vi "Measurement Logic.vi"() -> ()   [LabVIEW 2021, in "Short-Circuit.lvlib"]
uses:
  Short-Circuit.lvlib
  <instrlib>/niDCPower/nidcpower.llb/niDCPower Source Mode.ctl
  <instrlib>/niDCPower/nidcpower.llb/niDCPower Wait For Event - Event.ctl
  <instrlib>/niDCPower/nidcpower.llb/niDCPower Get Channel Name From String.vi
  Controls/LED_SCT_Data.ctl
  <instrlib>/niSwitch/niSwitch.llb/niSwitch Relay Action.ctl
  <instrlib>/niDMM/nidmm.llb/niDMM Function.ctl
  <instrlib>/niDMM/nidmm.llb/niDMM Configure Measurement Digits.vi
  <instrlib>/niDCPower/nidcpower.llb/niDCPower Output Function.ctl
  Measurement Results.ctl
  <instrlib>/niDCPower/nidcpower.llb/niDCPower Configure Digital Edge Source Trigger With Channels.vi
  <instrlib>/niDCPower/nidcpower.llb/niDCPower Configure Digital Edge Measure Trigger With Channels.vi
  <vilib>/Plug-In SDKs/Measurements/Measure Call Context/Measure Call Context.lvclass
  Measurement Configuration.ctl
panel:
  out "measurement results":T1={"Status"="Empty", "Source voltages"=[0.0], "Load voltages"=[0.0], "Source Current"=[0.0], "Load Current"=[0.0]}
  in  "measurement configuration":T2={"DUT setup time"=0.5, "Source delay"=0.5, "Aperture time"=0.5, "Source resource name"="Lorem ipsum dolor sit", "Source sense"=64, "Source current limit"=2.0, "Source maximum power"=20.0, "Source Voltage (Vo)"=3.5, "Load resource name"="", "Load sense"=-64, "Load voltage limit range"=60.0, "Load Voltage Limit"=6.0, "Load Current Level (Io)"=0.1, "Switch resource name"="", "Switch - Load Relay Name"="", "Switch - DMM Relay Name"="", "Relay Topology"="Configured Topology", "DMM resource name"="", "DMM Current Range(A)"=3.0, "SC - Trigger Delay (sec)"=5.0, "SC - Hold Delay (sec)"=5.0, "Resolution in Digits"=6.5} {"Resolution in Digits" items=["3 1/2"=3.5, "4 1/2"=4.5, "5 1/2"=5.5, "6 1/2"=6.5, "7 1/2"=7.5]; "Load Current Level (Io)" format="%.3f"; "Source Voltage (Vo)" format="%.2f"; "Load sense" items=["Local"=1008, "Remote"=1009]; "Source sense" items=["Local"=1008, "Remote"=1009]; "Aperture time" format="%#_6p"; "Source delay" format="%#_6p"; "DUT setup time" format="%#_6p"}
  out "measure call context out":refnum<class "Measure Call Context.lvclass">
  in  "measure call context in":refnum<class "Measure Call Context.lvclass">
  out "error out":errorcluster
  in  "error in":errorcluster
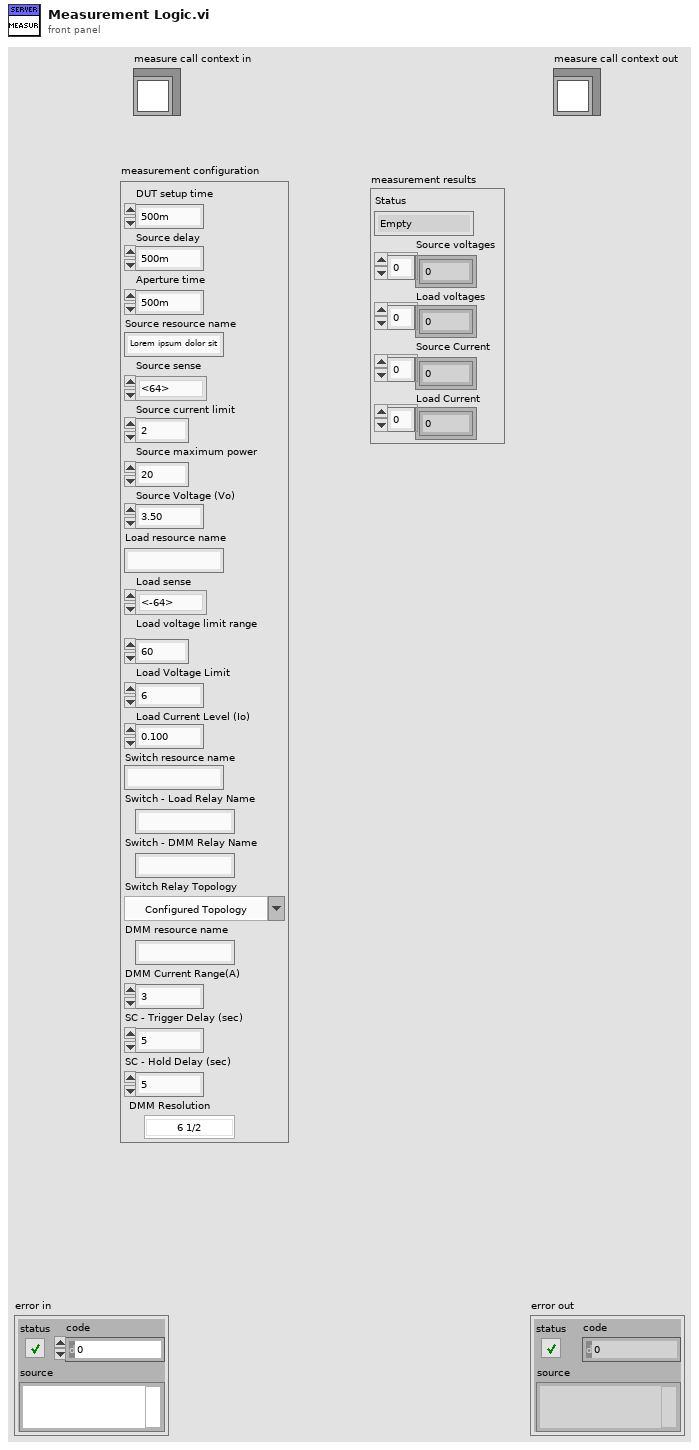
[diagram p1: front panel]
types:
  T1 = typedef "Short-Circuit.lvlib/Measurement Results.ctl" = cluster{"Status":string, "Source voltages":dbl[], "Load voltages":dbl[], "Source Current":dbl[], "Load Current":dbl[]}
  T2 = typedef "Short-Circuit.lvlib/Measurement Configuration.ctl" = cluster{"DUT setup time":dbl, "Source delay":dbl, "Aperture time":dbl, "Source resource name":string, "Source sense":i32, "Source current limit":dbl, "Source maximum power":dbl, "Source Voltage (Vo)":dbl, "Load resource name":string, "Load sense":i32, "Load voltage limit range":dbl, "Load Voltage Limit":dbl, "Load Current Level (Io)":dbl, "Switch resource name":string, "Switch - Load Relay Name":string, "Switch - DMM Relay Name":string, "Relay Topology":string, "DMM resource name":string, "DMM Current Range(A)":dbl, "SC - Trigger Delay (sec)":dbl, "SC - Hold Delay (sec)":dbl, "Resolution in Digits":dbl}
  T3 = typedef "Short-Circuit.lvlib/LED_SCT_Data.ctl" = cluster{"Load channel name":string, "Load out":refnum<k15>, "Source out":refnum<k15>, "Source channel name":string, "Source sequence name":string, "Source terminal name":string, "Measure terminal name":string, "Load Voltage-out":dbl[], "Load Current - out":dbl[], "Source Voltage-out":dbl[], "Source Current - out":dbl[], "Load Relay name":string, "DMM Relay name":string, "Switch out":refnum<k15>, "DMM out":refnum<k15>, "measurement results":T1, "SCT Completed?":bool, "DMM Current Reading":dbl}
  T4 = typedef "niDMM Function.ctl" = enum16{"DC Volts", "AC Volts", "DC Current", "AC Current", "2-wire Resistance", "4-wire Resistance", "Diode", "Frequency", "Period", "AC Volts DC Coupled", "Capacitance", "Inductance", "Temperature"}
  T5 = typedef "niDCPower Wait For Event - Event.ctl" = i32
  T6 = typedef "niDCPower Source Mode.ctl" = i32
  T7 = typedef "niSwitch Relay Action.ctl" = i32
  T8 = typedef "niDCPower Output Function.ctl" = i32
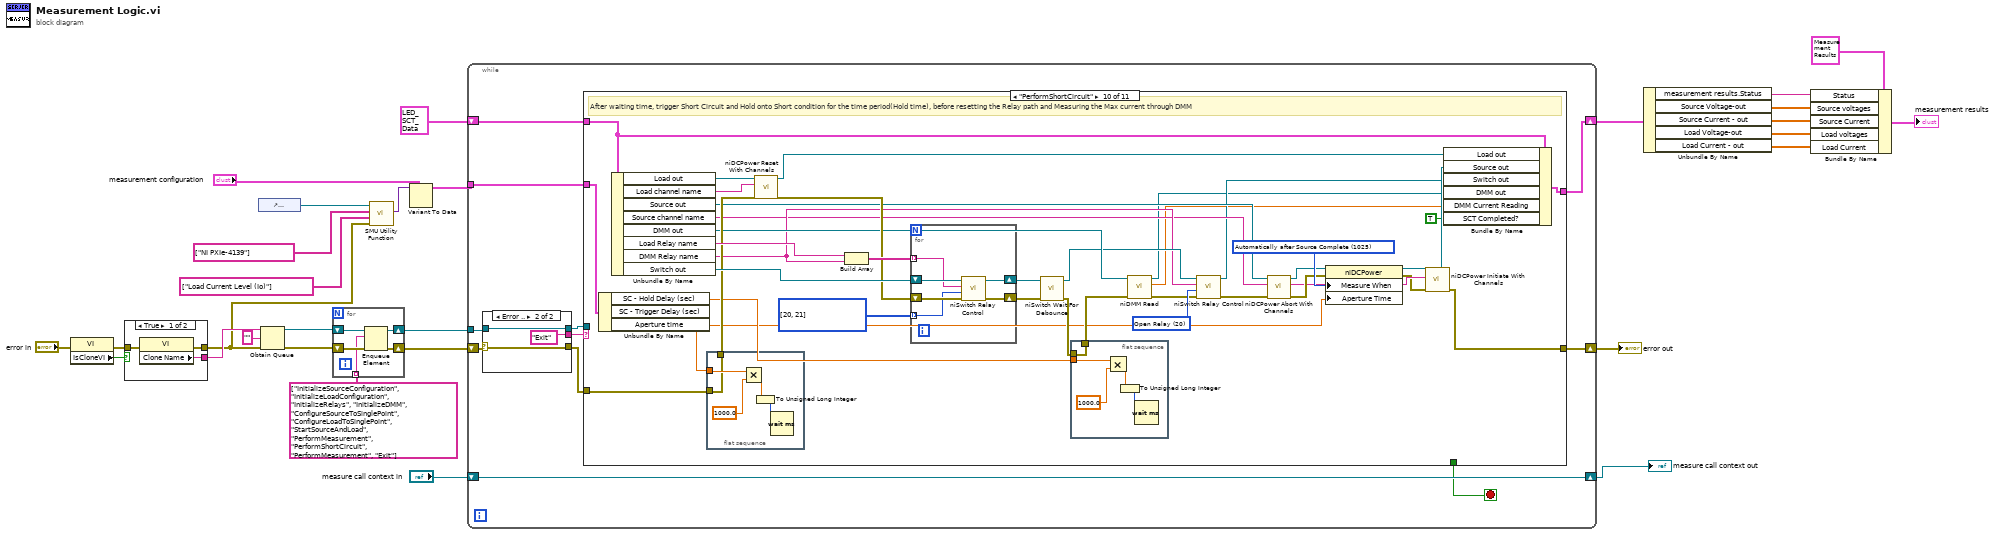
[diagram p0: block diagram]
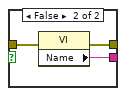
[diagram p2: hidden frame]
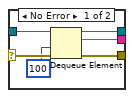
[diagram p3: hidden frame]
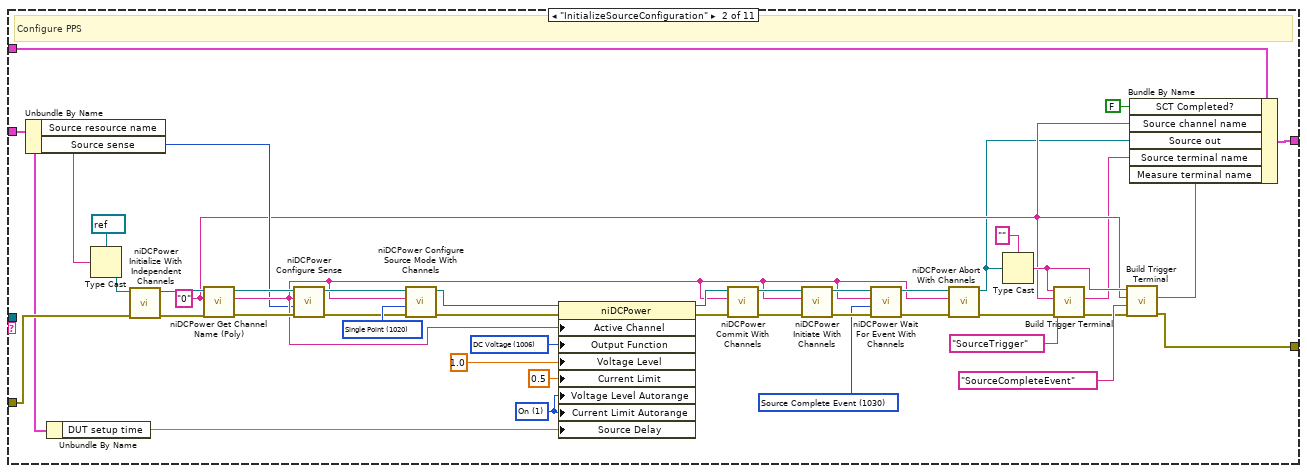
[diagram p5: hidden frame]
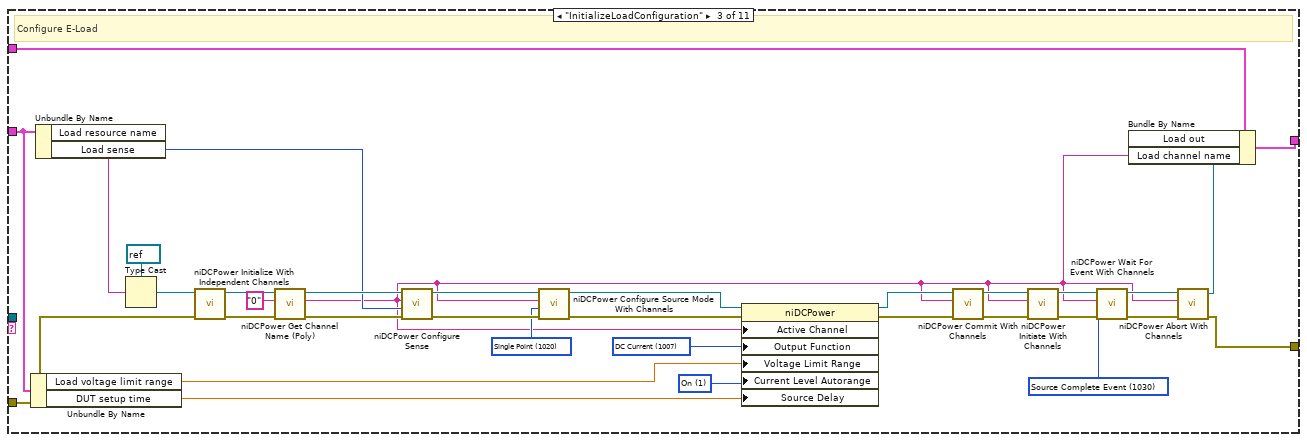
[diagram p6: hidden frame]
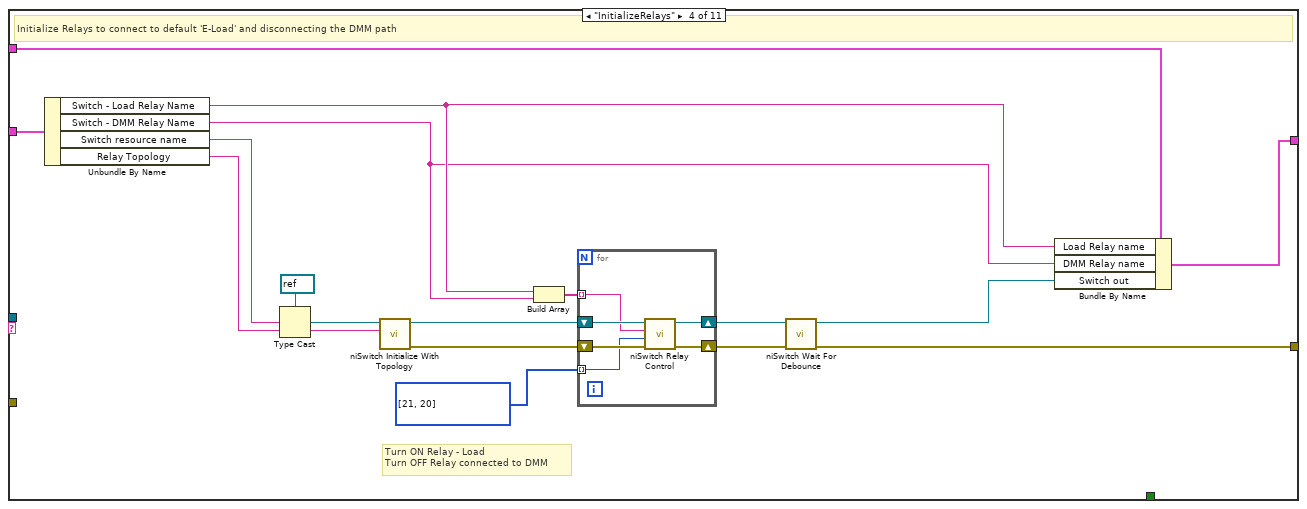
[diagram p7: hidden frame]
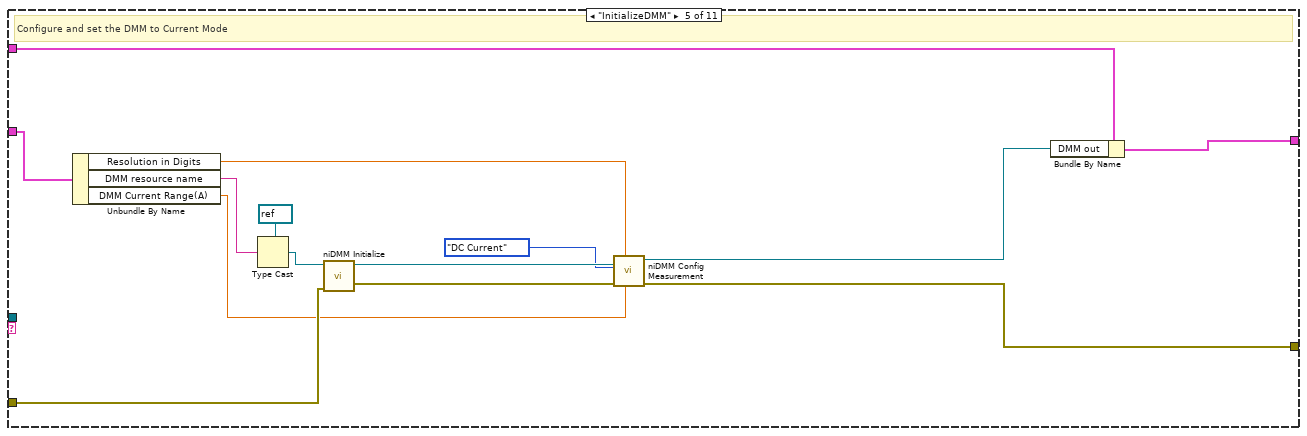
[diagram p8: hidden frame]
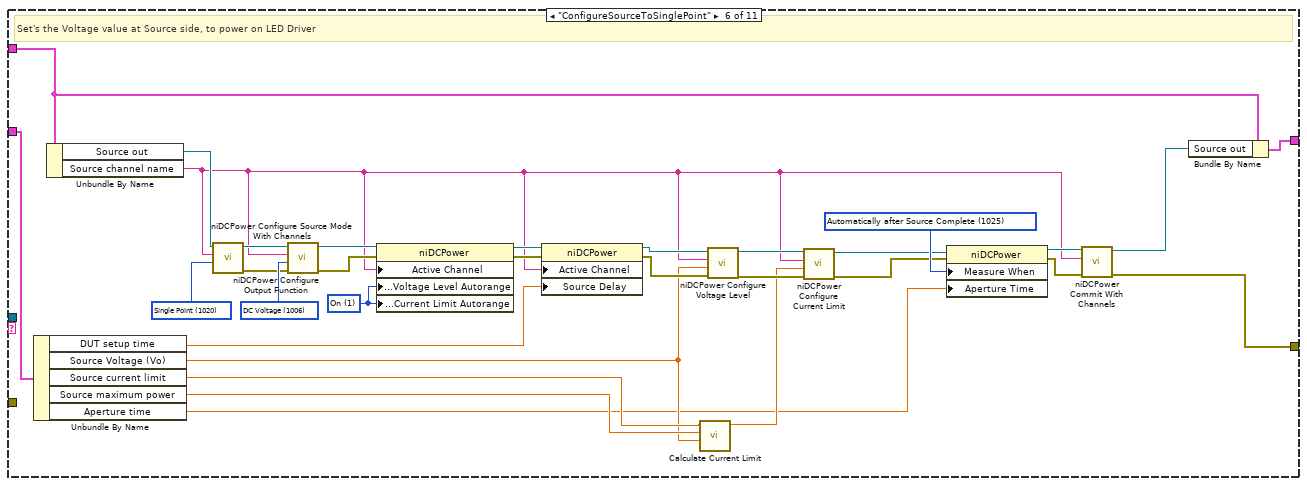
[diagram p9: hidden frame]
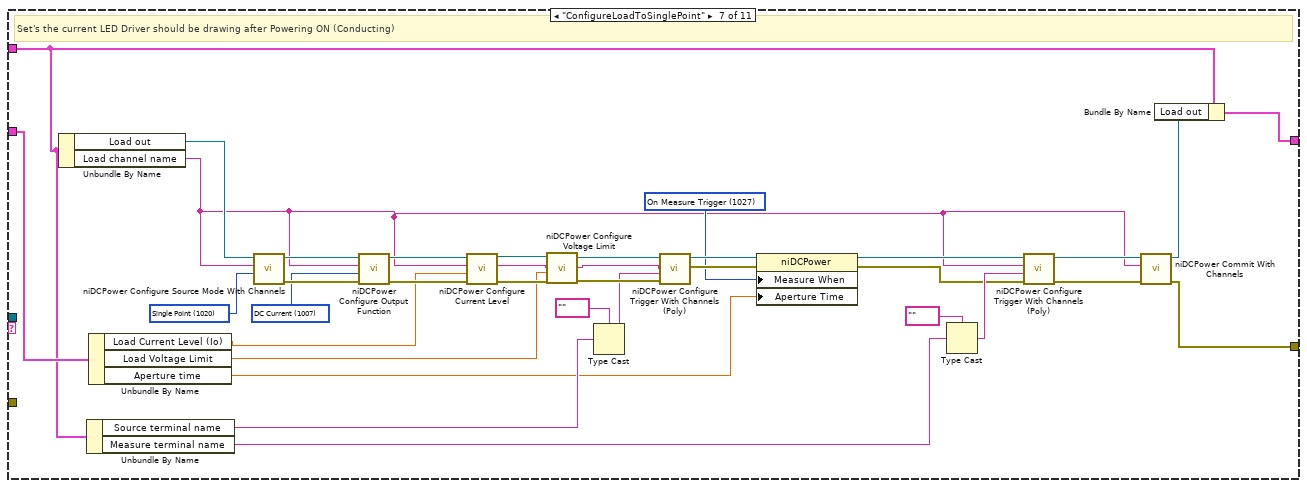
[diagram p10: hidden frame]
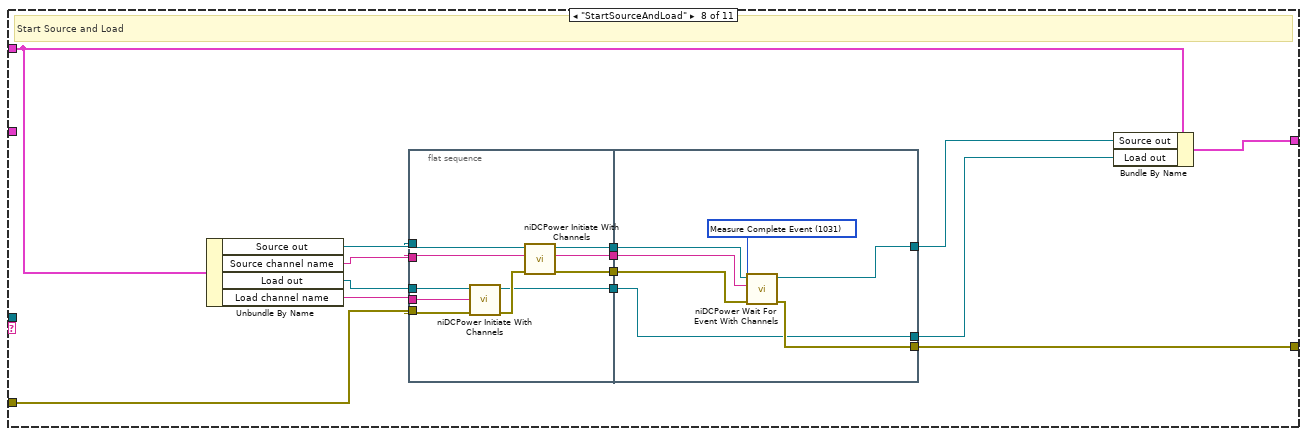
[diagram p11: hidden frame]
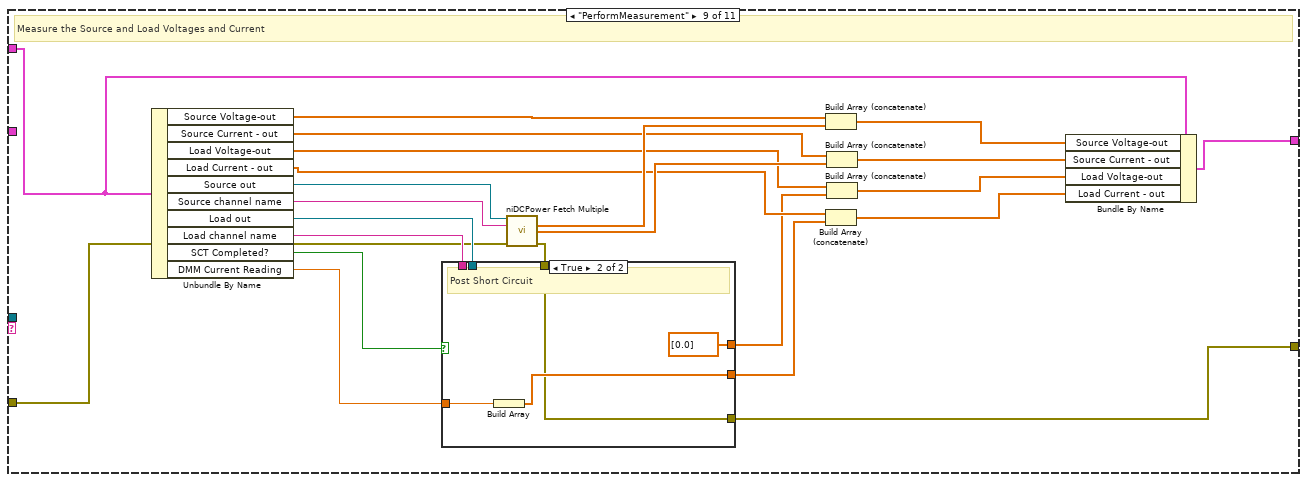
[diagram p12: hidden frame]
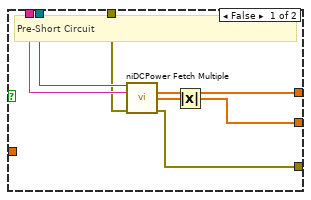
[diagram p13: hidden frame]
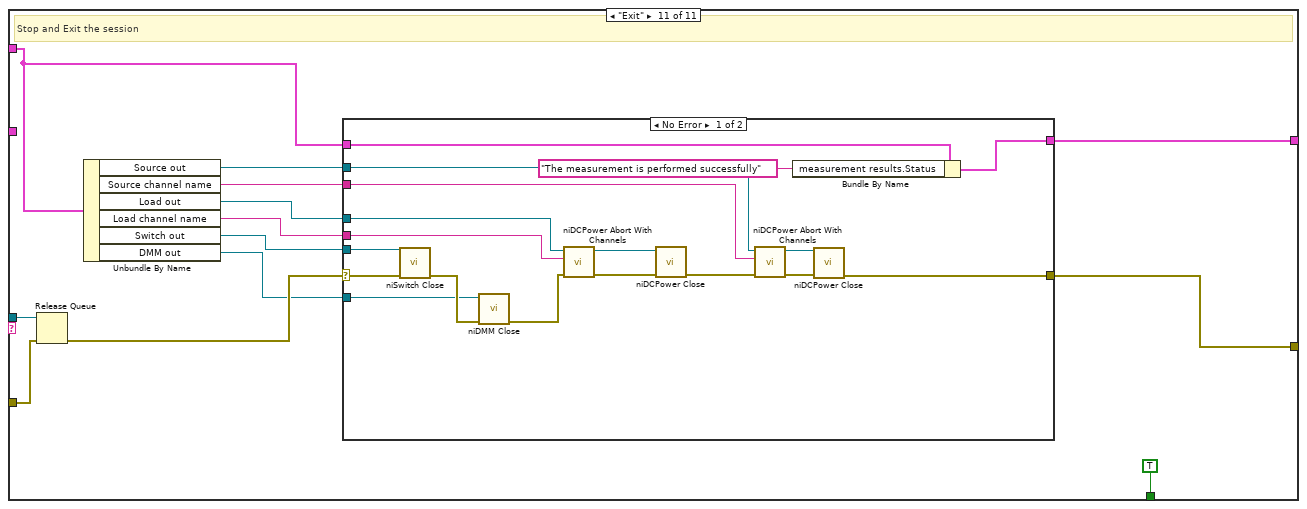
[diagram p14: hidden frame]
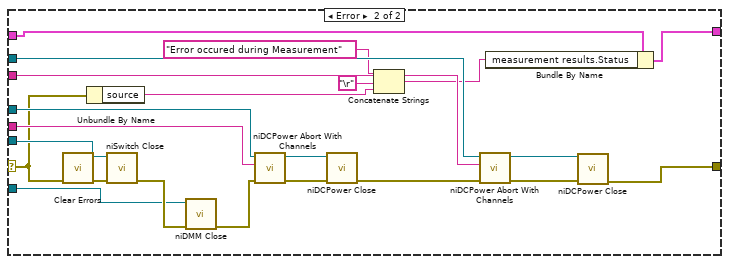
[diagram p15: hidden frame]
diagram:
  n1 = property class="VI"(error in="error in") -> (error out=w28:errorcluster, "IsCloneVI"=w29:bool)  [unwired: 1 in, 1 out]
  n2 = case shown="True" w29 {
    tunnel: [w32 w35] -> w4
    tunnel: [w31 w34] -> w23
    tunnel: w28 -> [w30 w33]
    frame True {
      n3 = property class="VI"(error in=w30) -> (error out=w32:errorcluster, "Clone Name"=w31:string)  [unwired: 1 in, 1 out]
    }
    frame False {
      n4 = property class="VI"(error in=w33) -> (error out=w35:errorcluster, "Name"=w34:string)  [unwired: 1 in, 1 out]
    }
  }
  n5 = control-ref of="measurement configuration"() -> (w7:refnum<vi>)
  n6 = Obtain Queue(name (unnamed)=w23, element data type="", error in (no error)=w4) -> (queue out=w26:refnum<queue>, error out=w27:errorcluster)  [unwired: 2 in, 1 out]
  n7 = for {
    shift-right: [w38] -> w21
    shift-left: w26 -> [w40]
    shift-right: [w37] -> w22
    shift-left: w27 -> [w39]
    tunnel: string[] ["InitializeSourceConfiguration", "InitializeLoadConfiguration", "InitializeRelays", "InitializeDMM", "ConfigureSourceToSinglePoint", "ConfigureLoadToSinglePoint", "StartSourceAndLoad", "PerformMeasurement", "PerformShortCircuit", "PerformMeasurement", "Exit"] ("Step sequence") -> [w36] mode=indexing
    n8 = Enqueue Element(queue=w40, element=w36, error in (no error)=w39) -> (queue out=w38:refnum<queue>, error out=w37:errorcluster)  [unwired: 1 in, 1 out]
  }
  n9 = call "SMU Utility Function.vi"("error in"=w4, "Load Current Parameters"=string[] ["Load Current Level (Io)"], "SMU Model"=string[] ["NI PXIe-4139"], "Measurement Configuration Ref"=w7) -> ("Measurement Configuration Out"=w3:variant)  [unwired: 6 in, 1 out]
  n10 = Variant To Data(type="measurement configuration", Variant=w3) -> (data=w1:T2)  [unwired: 1 in, 1 out]
  n11 = while {
    tunnel: w21 -> [w51]
    shift-right: [w44] -> w16
    shift-left: w22 -> [w50]
    tunnel: w1 -> [w47]
    shift-right: [w45] -> w15
    shift-left: T3 {"Load channel name"="", "Load out"="", "Source out"="", "Source channel name"="", "Source sequence name"="", "Source terminal name"="", "Measure terminal name"="", "Load Voltage-out"=[], "Load Current - out"=[], "Source Voltage-out"=[], "Source Current - out"=[], "Load Relay name"="", "DMM Relay name"="", "Switch out"="", "DMM out"="", "measurement results"={"Status"="Empty", "Source voltages"=[0.0], "Load voltages"=[0.0], "Source Current"=[0.0], "Load Current"=[0.0]}, "SCT Completed?"=FALSE, "DMM Current Reading"=0.0} ("Cluster") -> [w46]
    shift-right: [w43] -> w17
    shift-left: "measure call context in" -> [w43]
    stop <- w41 stop-if-true
    n12 = case shown="Error .." w50 {
      selector: w50 -> [w55 w59]
      tunnel: w51 -> [w57 w58]
      tunnel: [w56 "Exit" ("t")] -> w48
      tunnel: [w54 w59] -> w49
      tunnel: [w52 w58] -> w42
      frame No Error {
        n13 = Dequeue Element(queue=w57, timeout in ms (-1)=100, error in (no error)=w55) -> (queue out=w52:refnum<queue>, element=w56:string, error out=w54:errorcluster)  [unwired: 1 out]
      }
      frame Error {
      }
    }
    n14 = case shown="\"PerformShortCircuit\"" w48 {
      tunnel: w49 -> [w62 w83 w116 _ w170 _ _ w247 w275 w333 w372]
      tunnel: w47 -> [_ w78 w114 w151 w174 w184 w218 _ _ w334 _]
      tunnel: w46 -> [w61 w72 w112 w146 w167 w189 w212 w246 w281 w342 w370]
      tunnel: [w61 w67 w108 w142 w165 w187 w209 w243 w276 w306 w365] -> w45
      tunnel: [w62 w64 w109 w141 w164 w186 w210 w242 w273 w312 w364] -> w44
      tunnel: w42 -> [_ _ _ _ _ _ _ _ _ _ w373]
      tunnel: [_ _ _ _ _ _ _ _ _ _ TRUE] -> w41
      frame "", Default {
      }
      frame "InitializeSourceConfiguration" {
        w71 = "0" ("index")
        w90 = 1 items=["Off", "On"] ("Source:DC Voltage:Voltage Level Autorange")
        w91 = T5 1030 items=["Source Complete Event"=1030, "Measure Complete Event"=1031, "Sequence Iteration Complete Event"=1032, "Sequence Engine Done Event"=1033, "Pulse Complete Event"=1051, "Ready For Pulse Trigger Event"=1052] ("event")
        w102 = T6 1020 items=["Single Point"=1020, "Sequence"=1021] ("source mode")
        w97 = 1006 items=["DC Voltage"=1006, "DC Current"=1007, "Pulse Voltage"=1049, "Pulse Current"=1050] ("Source:Output Function")
        # "Configure PPS"
        n15 = Unbundle By Name(w78) -> ("Source resource name"=w81:string, "Source sense"=w79:i32)
        n16 = Unbundle By Name(w78) -> ("DUT setup time"=w77:dbl)
        n17 = Type Cast(type=refnum<k15> refnum ("resource name"), x=w81) -> (*(type *) &x=w80:refnum<k15>)
        n18 = call <instrlib>:"niDCPower Initialize With Independent Channels.vi"("error in (no error)"=w83, "resource name"=w80) -> ("error out"=w88:errorcluster, "instrument handle out"=w92:refnum<k15>)  [unwired: 8 in]
        n19 = call-poly <instrlib>:"niDCPower Get Channel Name (Poly).vi"("error in (no error)"=w88, "index"=w71, "instrument handle"=w92) -> ("error out"=w87:errorcluster, "name"=w84:string, "instrument handle out"=w89:refnum<k15>)  [unwired: 6 in]
        n20 = call <instrlib>:"niDCPower Configure Sense.vi"("error in (no error)"=w87, "sense"=w79, "channel name"=w84, "instrument handle"=w89) -> ("error out"=w100:errorcluster, "instrument handle out"=w98:refnum<k15>)  [unwired: 6 in]
        n21 = call <instrlib>:"niDCPower Configure Source Mode With Channels.vi"("error in (no error)"=w100, "source mode"=w102, "channel name"=w84, "instrument handle"=w98) -> ("error out"=w101:errorcluster, "instrument handle out"=w99:refnum<k15>)  [unwired: 6 in]
        n22 = property class="niDCPower"(reference=w99, error in=w101, "Active Channel"=w84, "Output Function"=w97, "Voltage Level"=1.0 ("Source:DC Voltage:Voltage Level"), "Current Limit"=0.5 ("Source:DC Voltage:Current Limit"), "Voltage Level Autorange"=w90, "Current Limit Autorange"=w90, "Source Delay"=w77) -> (reference out=w103:refnum<k15>, error out=w104:errorcluster)
        n23 = call <instrlib>:"niDCPower Commit With Channels.vi"("error in (no error)"=w104, "channel name"=w84, "instrument handle"=w103) -> ("error out"=w106:errorcluster, "instrument handle out"=w105:refnum<k15>)  [unwired: 7 in]
        n24 = call <instrlib>:"niDCPower Initiate With Channels.vi"("error in (no error)"=w106, "channel name"=w84, "instrument handle"=w105) -> ("error out"=w93:errorcluster, "instrument handle out"=w94:refnum<k15>)  [unwired: 7 in]
        n25 = call <instrlib>:"niDCPower Wait For Event With Channels.vi"("error in (no error)"=w93, "event"=w91, "channel name"=w84, "instrument handle"=w94) -> ("error out"=w96:errorcluster, "instrument handle out"=w95:refnum<k15>)  [unwired: 6 in]
        n26 = call <instrlib>:"niDCPower Abort With Channels.vi"("error in (no error)"=w96, "channel name"=w84, "instrument handle"=w95) -> ("error out"=w66:errorcluster, "instrument handle out"=w70:refnum<k15>)  [unwired: 7 in]
        n27 = Type Cast(type="", x=w70) -> (*(type *) &x=w75:string)
        n28 = call "Build Trigger Terminal.vi"("error in (no error)"=w66, "Trigger/Event Name"="SourceTrigger", "Channel Name"=w71, "Resource Name"=w75) -> ("error out"=w65:errorcluster, "Terminal Name"=w69:string)  [unwired: 6 in]
        n29 = call "Build Trigger Terminal.vi"("error in (no error)"=w65, "Trigger/Event Name"="SourceCompleteEvent", "Channel Name"=w71, "Resource Name"=w75) -> ("error out"=w64:errorcluster, "Terminal Name"=w68:string)  [unwired: 6 in]
        n30 = Bundle By Name(cluster=w72, "SCT Completed?"=FALSE, "Source channel name"=w71, "Source out"=w70, "Source terminal name"=w69, "Measure terminal name"=w68) -> (w67:T3)
      }
      frame "InitializeLoadConfiguration" {
        w121 = T6 1020 items=["Single Point"=1020, "Sequence"=1021] ("source mode")
        w122 = T5 1030 items=["Source Complete Event"=1030, "Measure Complete Event"=1031, "Sequence Iteration Complete Event"=1032, "Sequence Engine Done Event"=1033, "Pulse Complete Event"=1051, "Ready For Pulse Trigger Event"=1052] ("event")
        w123 = 1 items=["Off", "On"] ("Source:DC Current:Current Level Autorange")
        w124 = 1007 items=["DC Voltage"=1006, "DC Current"=1007, "Pulse Voltage"=1049, "Pulse Current"=1050] ("Source:Output Function")
        # "Configure E-Load"
        n31 = Unbundle By Name(w114) -> ("Load voltage limit range"=w107:dbl, "DUT setup time"=w113:dbl)
        n32 = Unbundle By Name(w114) -> ("Load resource name"=w118:string, "Load sense"=w115:i32)
        n33 = Type Cast(type=refnum<k15> refnum ("resource name"), x=w118) -> (*(type *) &x=w117:refnum<k15>)
        n34 = call <instrlib>:"niDCPower Initialize With Independent Channels.vi"("error in (no error)"=w116, "resource name"=w117) -> ("error out"=w139:errorcluster, "instrument handle out"=w137:refnum<k15>)  [unwired: 8 in]
        n35 = call-poly <instrlib>:"niDCPower Get Channel Name (Poly).vi"("error in (no error)"=w139, "index"="0", "instrument handle"=w137) -> ("error out"=w140:errorcluster, "name"=w110:string, "instrument handle out"=w138:refnum<k15>)  [unwired: 6 in]
        n36 = call <instrlib>:"niDCPower Configure Sense.vi"("error in (no error)"=w140, "sense"=w115, "channel name"=w110, "instrument handle"=w138) -> ("error out"=w131:errorcluster, "instrument handle out"=w132:refnum<k15>)  [unwired: 6 in]
        n37 = call <instrlib>:"niDCPower Configure Source Mode With Channels.vi"("error in (no error)"=w131, "source mode"=w121, "channel name"=w110, "instrument handle"=w132) -> ("error out"=w129:errorcluster, "instrument handle out"=w130:refnum<k15>)  [unwired: 6 in]
        n38 = property class="niDCPower"(reference=w130, error in=w129, "Active Channel"=w110, "Output Function"=w124, "Voltage Limit Range"=w107, "Current Level Autorange"=w123, "Source Delay"=w113) -> (reference out=w128:refnum<k15>, error out=w127:errorcluster)
        n39 = call <instrlib>:"niDCPower Commit With Channels.vi"("error in (no error)"=w127, "channel name"=w110, "instrument handle"=w128) -> ("error out"=w126:errorcluster, "instrument handle out"=w125:refnum<k15>)  [unwired: 7 in]
        n40 = call <instrlib>:"niDCPower Initiate With Channels.vi"("error in (no error)"=w126, "channel name"=w110, "instrument handle"=w125) -> ("error out"=w136:errorcluster, "instrument handle out"=w135:refnum<k15>)  [unwired: 7 in]
        n41 = call <instrlib>:"niDCPower Wait For Event With Channels.vi"("error in (no error)"=w136, "event"=w122, "channel name"=w110, "instrument handle"=w135) -> ("error out"=w133:errorcluster, "instrument handle out"=w134:refnum<k15>)  [unwired: 6 in]
        n42 = call <instrlib>:"niDCPower Abort With Channels.vi"("error in (no error)"=w133, "channel name"=w110, "instrument handle"=w134) -> ("error out"=w109:errorcluster, "instrument handle out"=w111:refnum<k15>)  [unwired: 7 in]
        n43 = Bundle By Name(cluster=w112, "Load out"=w111, "Load channel name"=w110) -> (w108:T3)
      }
      frame "InitializeRelays" {
        w154 = T7[] [21, 20] items=["Open Relay"=20, "Close Relay"=21]
        # "Turn ON Relay - Load\nTurn OFF Relay connected to DMM"
        # "Initialize Relays to connect to default 'E-Load' and disconnecting the DMM path"
        n44 = Unbundle By Name(w151) -> ("Switch - Load Relay Name"=w144:string, "Switch - DMM Relay Name"=w143:string, "Switch resource name"=w149:string, "Relay Topology"=w147:string)
        n45 = Type Cast(type=refnum<k15> refnum ("resource name"), x=w149) -> (*(type *) &x=w148:refnum<k15>)
        n46 = call <instrlib>:"niSwitch Initialize With Topology.vi"("topology name"=w147, "resource name"=w148) -> ("error out"=w156:errorcluster, "instrument handle out"=w157:refnum<k15>)  [unwired: 3 in, 5 out]
        n47 = Build Array(w144, w143) -> (w155:string[])
        n48 = for {
          tunnel: w155 -> [w161] mode=indexing
          tunnel: w154 -> [w160] mode=indexing
          shift-right: [w158] -> w152
          shift-left: w156 -> [w162]
          shift-right: [w159] -> w153
          shift-left: w157 -> [w163]
          n49 = call <instrlib>:"niSwitch Relay Control.vi"("error in (no error)"=w162, "relay action (Close Relay)"=w160, "relay names"=w161, "instrument handle"=w163) -> ("error out"=w158:errorcluster, "instrument handle out"=w159:refnum<k15>)  [unwired: 6 out]
        }
        n50 = call <instrlib>:"niSwitch Wait For Debounce.vi"("error in (no error)"=w152, "instrument handle"=w153) -> ("error out"=w141:errorcluster, "instrument handle out"=w145:refnum<k15>)  [unwired: 1 in, 7 out]
        n51 = Bundle By Name(cluster=w146, "Load Relay name"=w144, "DMM Relay name"=w143, "Switch out"=w145) -> (w142:T3)
      }
      frame "InitializeDMM" {
        # "Configure and set the DMM to Current Mode"
        n52 = Unbundle By Name(w174) -> ("Resolution in Digits"=w169:dbl, "DMM resource name"=w172:string, "DMM Current Range(A)"=w168:dbl)
        n53 = Type Cast(type=refnum<k15> refnum ("resource name"), x=w172) -> (*(type *) &x=w171:refnum<k15>)
        n54 = call <instrlib>:"niDMM Initialize.vi"("error in (no error)"=w170, "Instrument Descriptor"=w171) -> ("error out"=w175:errorcluster, "instrument handle out"=w177:refnum<k15>)  [unwired: 8 in]
        n55 = call-poly <instrlib>:"niDMM Config Measurement.vi"("Range"=w168, "Resolution in Digits"=w169, "error in (no error)"=w175, "Function"=niDMM_Function."DC Current", "instrument handle"=w177) -> ("error out"=w164:errorcluster, "instrument handle out"=w166:refnum<k15>)  [unwired: 5 in]
        n56 = Bundle By Name(cluster=w167, "DMM out"=w166) -> (w165:T3)
      }
      frame "ConfigureSourceToSinglePoint" {
        w199 = 1025 items=["Automatically after Source Complete"=1025, "On Demand"=1026, "On Measure Trigger"=1027] ("Measurement:Advanced:Measure When")
        w204 = 1 items=["Off", "On"] ("DC Voltage:Voltage Level Autorange")
        w203 = T8 1006 items=["DC Voltage"=1006, "DC Current"=1007, "Pulse Voltage"=1049, "Pulse Current"=1050] ("output function")
        w202 = T6 1020 items=["Single Point"=1020, "Sequence"=1021] ("source mode")
        # "Set's the Voltage value at Source side, to power on LED Driver"
        n57 = Unbundle By Name(w184) -> ("DUT setup time"=w183:dbl, "Source Voltage (Vo)"=w180:dbl, "Source current limit"=w182:dbl, "Source maximum power"=w181:dbl, "Aperture time"=w178:dbl)
        n58 = Unbundle By Name(w189) -> ("Source out"=w190:refnum<k15>, "Source channel name"=w185:string)
        n59 = call <instrlib>:"niDCPower Configure Source Mode With Channels.vi"("source mode"=w202, "channel name"=w185, "instrument handle"=w190) -> ("error out"=w200:errorcluster, "instrument handle out"=w201:refnum<k15>)  [unwired: 7 in]
        n60 = call <instrlib>:"niDCPower Configure Output Function.vi"("error in (no error)"=w200, "output function"=w203, "channel name"=w185, "instrument handle"=w201) -> ("error out"=w208:errorcluster, "instrument handle out"=w207:refnum<k15>)  [unwired: 6 out]
        n61 = property class="niDCPower"(reference=w207, error in=w208, "Active Channel"=w185, "Source:DC Voltage:Voltage Level Autorange"=w204, "Source:DC Voltage:Current Limit Autorange"=w204) -> (reference out=w205:refnum<k15>, error out=w206:errorcluster)
        n62 = property class="niDCPower"(reference=w205, error in=w206, "Active Channel"=w185, "Source Delay"=w183) -> (reference out=w196:refnum<k15>, error out=w195:errorcluster)
        n63 = call "Calculate Current Limit.vi"("Voltage value"=w180, "Maximum power"=w181, "Current limit in"=w182) -> ("Current limit out"=w179:dbl)  [unwired: 8 in]
        n64 = call <instrlib>:"niDCPower Configure Voltage Level.vi"("error in (no error)"=w195, "voltage level"=w180, "channel name"=w185, "instrument handle"=w196) -> ("error out"=w193:errorcluster, "instrument handle out"=w194:refnum<k15>)  [unwired: 6 in]
        n65 = call <instrlib>:"niDCPower Configure Current Limit.vi"("error in (no error)"=w193, "current limit"=w179, "channel name"=w185, "instrument handle"=w194) -> ("error out"=w191:errorcluster, "instrument handle out"=w192:refnum<k15>)  [unwired: 6 in]
        n66 = property class="niDCPower"(reference=w192, error in=w191, "Measure When"=w199, "Aperture Time"=w178) -> (reference out=w197:refnum<k15>, error out=w198:errorcluster)
        n67 = call <instrlib>:"niDCPower Commit With Channels.vi"("error in (no error)"=w198, "channel name"=w185, "instrument handle"=w197) -> ("error out"=w186:errorcluster, "instrument handle out"=w188:refnum<k15>)  [unwired: 7 in]
        n68 = Bundle By Name(cluster=w189, "Source out"=w188) -> (w187:T3)
      }
      frame "ConfigureLoadToSinglePoint" {
        w223 = T8 1007 items=["DC Voltage"=1006, "DC Current"=1007, "Pulse Voltage"=1049, "Pulse Current"=1050] ("output function")
        w225 = 1027 items=["Automatically after Source Complete"=1025, "On Demand"=1026, "On Measure Trigger"=1027] ("Measurement:Advanced:Measure When")
        w224 = T6 1020 items=["Single Point"=1020, "Sequence"=1021] ("source mode")
        # "Set's the current LED Driver should be drawing after Powering ON (Conducting)"
        n69 = Unbundle By Name(w212) -> ("Load out"=w220:refnum<k15>, "Load channel name"=w219:string)
        n70 = Unbundle By Name(w212) -> ("Source terminal name"=w215:string, "Measure terminal name"=w214:string)
        n71 = Unbundle By Name(w218) -> ("Load Current Level (Io)"=w217:dbl, "Load Voltage Limit"=w216:dbl, "Aperture time"=w213:dbl)
        n72 = call <instrlib>:"niDCPower Configure Source Mode With Channels.vi"("source mode"=w224, "channel name"=w219, "instrument handle"=w220) -> ("error out"=w230:errorcluster, "instrument handle out"=w229:refnum<k15>)  [unwired: 7 in]
        n73 = call <instrlib>:"niDCPower Configure Output Function.vi"("error in (no error)"=w230, "output function"=w223, "channel name"=w219, "instrument handle"=w229) -> ("error out"=w236:errorcluster, "instrument handle out"=w237:refnum<k15>)  [unwired: 6 in]
        n74 = call <instrlib>:"niDCPower Configure Current Level.vi"("error in (no error)"=w236, "current level"=w217, "channel name"=w219, "instrument handle"=w237) -> ("error out"=w238:errorcluster, "instrument handle out"=w241:refnum<k15>)  [unwired: 6 in]
        n75 = call <instrlib>:"niDCPower Configure Voltage Limit.vi"("error in (no error)"=w238, "voltage limit"=w216, "channel name"=w219, "instrument handle"=w241) -> ("error out"=w239:errorcluster, "instrument handle out"=w240:refnum<k15>)  [unwired: 6 in]
        n76 = Type Cast(type=tag "" ("input terminal"), x=w215) -> (*(type *) &x=w234:tag)
        n77 = call-poly <instrlib>:"niDCPower Configure Trigger With Channels (Poly).vi"("error in (no error)"=w239, "input terminal"=w234, "channel name"=w219, "instrument handle"=w240) -> ("error out"=w233:errorcluster, "instrument handle out"=w226:refnum<k15>)  [unwired: 6 in]
        n78 = property class="niDCPower"(reference=w226, error in=w233, "Measure When"=w225, "Aperture Time"=w213) -> (reference out=w231:refnum<k15>, error out=w232:errorcluster)
        n79 = Type Cast(type=tag "" ("input terminal"), x=w214) -> (*(type *) &x=w235:tag)
        n80 = call-poly <instrlib>:"niDCPower Configure Trigger With Channels (Poly).vi"("error in (no error)"=w232, "input terminal"=w235, "channel name"=w219, "instrument handle"=w231) -> ("error out"=w228:errorcluster, "instrument handle out"=w227:refnum<k15>)  [unwired: 6 in]
        n81 = call <instrlib>:"niDCPower Commit With Channels.vi"("error in (no error)"=w228, "channel name"=w219, "instrument handle"=w227) -> ("error out"=w210:errorcluster, "instrument handle out"=w211:refnum<k15>)  [unwired: 7 in]
        n82 = Bundle By Name(cluster=w212, "Load out"=w211) -> (w209:T3)
      }
      frame "StartSourceAndLoad" {
        # "Start Source and Load"
        n83 = Unbundle By Name(w246) -> ("Source out"=w251:refnum<k15>, "Source channel name"=w250:string, "Load out"=w249:refnum<k15>, "Load channel name"=w248:string)
        n84 = flat-sequence {
          tunnel: [w263] -> w255
          tunnel: [w262] -> w254
          tunnel: w247 -> [w261]
          tunnel: w249 -> [w260]
          tunnel: w251 -> [w259]
          tunnel: w250 -> [w257]
          tunnel: w248 -> [w256]
          tunnel: [w258] -> w253
          tunnel: [w257] -> w252
          tunnel: w255 -> [w269]
          tunnel: w254 -> [w266]
          tunnel: [w266] -> w244
          tunnel: w253 -> [w271]
          tunnel: w252 -> [w270]
          tunnel: [w268] -> w242
          tunnel: [w267] -> w245
          frame #0 {
            n85 = call <instrlib>:"niDCPower Initiate With Channels.vi"("error in (no error)"=w261, "channel name"=w256, "instrument handle"=w260) -> ("error out"=w264:errorcluster, "instrument handle out"=w262:refnum<k15>)  [unwired: 7 in]
            n86 = call <instrlib>:"niDCPower Initiate With Channels.vi"("error in (no error)"=w264, "channel name"=w257, "instrument handle"=w259) -> ("error out"=w263:errorcluster, "instrument handle out"=w258:refnum<k15>)  [unwired: 7 in]
          }
          frame #1 {
            w265 = T5 1031 items=["Source Complete Event"=1030, "Measure Complete Event"=1031, "Sequence Iteration Complete Event"=1032, "Sequence Engine Done Event"=1033, "Pulse Complete Event"=1051, "Ready For Pulse Trigger Event"=1052] ("event")
            n87 = call <instrlib>:"niDCPower Wait For Event With Channels.vi"("error in (no error)"=w269, "event"=w265, "channel name"=w270, "instrument handle"=w271) -> ("error out"=w268:errorcluster, "instrument handle out"=w267:refnum<k15>)  [unwired: 6 in]
          }
        }
        n88 = Bundle By Name(cluster=w246, "Source out"=w245, "Load out"=w244) -> (w243:T3)
      }
      frame "PerformMeasurement" {
        # "Measure the Source and Load Voltages and Current"
        n89 = Unbundle By Name(w281) -> ("Source Voltage-out"=w289:dbl[], "Source Current - out"=w287:dbl[], "Load Voltage-out"=w285:dbl[], "Load Current - out"=w284:dbl[], "Source out"=w294:refnum<k15>, "Source channel name"=w293:string, "Load out"=w292:refnum<k15>, "Load channel name"=w291:string, "SCT Completed?"=w290:bool, "DMM Current Reading"=w272:dbl)
        n90 = call <instrlib>:"niDCPower Fetch Multiple.vi"("instrument handle"=w294, "channel name"=w293, "error in (no error)"=w275) -> ("voltage measurements"=w288:dbl[], "current measurements"=w286:dbl[], "error out"=w274:errorcluster)  [unwired: 2 in, 8 out]
        n91 = case shown="True" w290 {
          tunnel: w292 -> [w301 _]
          tunnel: w291 -> [w300 _]
          tunnel: [w299 dbl[] [0.0] ("voltage measurements")] -> w283
          tunnel: [w295 w303] -> w282
          tunnel: w274 -> [w297 w302]
          tunnel: [w296 w302] -> w273
          tunnel: w272 -> [_ w304]
          frame False {
            # "Pre-Short Circuit"
            n92 = call <instrlib>:"niDCPower Fetch Multiple.vi"("instrument handle"=w301, "channel name"=w300, "error in (no error)"=w297) -> ("voltage measurements"=w299:dbl[], "current measurements"=w298:dbl[], "error out"=w296:errorcluster)  [unwired: 2 in, 8 out]
            n93 = Absolute Value(x=w298) -> (abs(x)=w295:dbl[])
          }
          frame True {
            # "Post Short Circuit"
            n94 = Build Array(w304) -> (w303:dbl[])
          }
        }
        n95 = Build Array (concatenate)(w289, w288) -> (w280:dbl[])
        n96 = Build Array (concatenate)(w284, w282) -> (w277:dbl[])
        n97 = Build Array (concatenate)(w287, w286) -> (w279:dbl[])
        n98 = Build Array (concatenate)(w285, w283) -> (w278:dbl[])
        n99 = Bundle By Name(cluster=w281, "Source Voltage-out"=w280, "Source Current - out"=w279, "Load Voltage-out"=w278, "Load Current - out"=w277) -> (w276:T3)
      }
      frame "PerformShortCircuit" {
        w319 = 1025 items=["Automatically after Source Complete"=1025, "On Demand"=1026, "On Measure Trigger"=1027] ("Measurement:Advanced:Measure When")
        w323 = T7 20 items=["Open Relay"=20, "Close Relay"=21] ("relay action (Close Relay)")
        w340 = T7[] [20, 21] items=["Open Relay"=20, "Close Relay"=21]
        # "After waiting time, trigger Short Circuit and Hold onto Short condition for the time period(Hold time), before resetting the Relay path and Measuring the Max current through DMM"
        n100 = Unbundle By Name(w334) -> ("SC - Hold Delay (sec)"=w328:dbl, "SC - Trigger Delay (sec)"=w327:dbl, "Aperture time"=w316:dbl)
        n101 = Unbundle By Name(w342) -> ("Load out"=w344:refnum<k15>, "Load channel name"=w343:string, "Source out"=w321:refnum<k15>, "Source channel name"=w314:string, "DMM out"=w326:refnum<k15>, "Load Relay name"=w336:string, "DMM Relay name"=w324:string, "Switch out"=w335:refnum<k15>)
        n102 = flat-sequence {
          tunnel: w327 -> [w354]
          tunnel: [w350] -> w332
          tunnel: w333 -> [w350]
          frame #0 {
            n103 = Multiply(x=w354, y=1000.0) -> (x*y=w352:dbl)
            n104 = To Unsigned Long Integer(number=w352) -> (unsigned 32bit integer=w351:u32)
            n105 = Wait (ms)(milliseconds to wait=w351) -> ()  [unwired: 1 out]
          }
        }
        n106 = call <instrlib>:"niDCPower Reset With Channels.vi"("error in (no error)"=w332, "channel name"=w343, "instrument handle"=w344) -> ("error out"=w331:errorcluster, "instrument handle out"=w341:refnum<k15>)  [unwired: 7 in]
        n107 = Build Array(w336, w324) -> (w339:string[])
        n108 = for {
          tunnel: w339 -> [w358] mode=indexing
          tunnel: w340 -> [w357] mode=indexing
          shift-right: [w355] -> w338
          shift-left: w331 -> [w359]
          shift-right: [w356] -> w337
          shift-left: w335 -> [w360]
          n109 = call <instrlib>:"niSwitch Relay Control.vi"("error in (no error)"=w359, "relay action (Close Relay)"=w357, "relay names"=w358, "instrument handle"=w360) -> ("error out"=w355:errorcluster, "instrument handle out"=w356:refnum<k15>)  [unwired: 6 out]
        }
        n110 = call <instrlib>:"niSwitch Wait For Debounce.vi"("error in (no error)"=w338, "instrument handle"=w337) -> ("error out"=w330:errorcluster, "instrument handle out"=w325:refnum<k15>)  [unwired: 1 in, 7 out]
        n111 = flat-sequence {
          tunnel: w328 -> [w349]
          tunnel: [w345] -> w329
          tunnel: w330 -> [w345]
          frame #0 {
            n112 = Multiply(x=w349, y=1000.0) -> (x*y=w347:dbl)
            n113 = To Unsigned Long Integer(number=w347) -> (unsigned 32bit integer=w346:u32)
            n114 = Wait (ms)(milliseconds to wait=w346) -> ()  [unwired: 1 out]
          }
        }
        n115 = call <instrlib>:"niDMM Read.vi"("error in (no error)"=w329, "instrument handle"=w326) -> ("error out"=w322:errorcluster, "Measurement"=w308:dbl, "instrument handle out"=w309:refnum<k15>)  [unwired: 7 in]
        n116 = call <instrlib>:"niSwitch Relay Control.vi"("error in (no error)"=w322, "relay action (Close Relay)"=w323, "relay names"=w324, "instrument handle"=w325) -> ("error out"=w320:errorcluster, "instrument handle out"=w310:refnum<k15>)  [unwired: 6 out]
        n117 = call <instrlib>:"niDCPower Abort With Channels.vi"("error in (no error)"=w320, "channel name"=w314, "instrument handle"=w321) -> ("error out"=w317:errorcluster, "instrument handle out"=w318:refnum<k15>)  [unwired: 7 in]
        n118 = property class="niDCPower"(reference=w318, error in=w317, "Measure When"=w319, "Aperture Time"=w316) -> (reference out=w315:refnum<k15>, error out=w313:errorcluster)
        n119 = call <instrlib>:"niDCPower Initiate With Channels.vi"("error in (no error)"=w313, "channel name"=w314, "instrument handle"=w315) -> ("error out"=w312:errorcluster, "instrument handle out"=w311:refnum<k15>)  [unwired: 7 in]
        n120 = Bundle By Name(cluster=w342, "Load out"=w341, "Source out"=w311, "Switch out"=w310, "DMM out"=w309, "DMM Current Reading"=w308, "SCT Completed?"=TRUE) -> (w306:T3)
      }
      frame "Exit" {
        # "Stop and Exit the session"
        n121 = Release Queue(queue=w373, error in (no error)=w372) -> (error out=w371:errorcluster)  [unwired: 1 in, 2 out]
        n122 = Unbundle By Name(w370) -> ("Source out"=w369:refnum<k15>, "Source channel name"=w368:string, "Load out"=w367:refnum<k15>, "Load channel name"=w366:string, "Switch out"=w363:refnum<k15>, "DMM out"=w362:refnum<k15>)
        n123 = case shown="No Error" w371 {
          selector: w371 -> [w376 w394]
          tunnel: w367 -> [w387 w410]
          tunnel: w366 -> [w388 w407]
          tunnel: w368 -> [w382 w406]
          tunnel: [w383 w409] -> w364
          tunnel: w369 -> [w384 w408]
          tunnel: w370 -> [w380 w405]
          tunnel: [w379 w404] -> w365
          tunnel: w363 -> [w377 w403]
          tunnel: w362 -> [w375 w400]
          frame No Error {
            n124 = call <instrlib>:"niSwitch Close.vi"("error in (no error)"=w376, "instrument handle"=w377) -> ("error out"=w378:errorcluster)  [unwired: 9 in]
            n125 = call <instrlib>:"niDMM Close.vi"("error in (no error)"=w378, "instrument handle"=w375) -> ("error out"=w374:errorcluster)  [unwired: 9 in]
            n126 = call <instrlib>:"niDCPower Abort With Channels.vi"("error in (no error)"=w374, "channel name"=w388, "instrument handle"=w387) -> ("error out"=w385:errorcluster, "instrument handle out"=w386:refnum<k15>)  [unwired: 7 in]
            n127 = call <instrlib>:"niDCPower Close.vi"("error in (no error)"=w385, "instrument handle"=w386) -> ("error out"=w389:errorcluster)  [unwired: 9 in]
            n128 = call <instrlib>:"niDCPower Abort With Channels.vi"("error in (no error)"=w389, "channel name"=w382, "instrument handle"=w384) -> ("error out"=w391:errorcluster, "instrument handle out"=w390:refnum<k15>)  [unwired: 7 in]
            n129 = Bundle By Name(cluster=w380, "measurement results.Status"="The measurement is performed successfully" ("message")) -> (w379:T3)
            n130 = call <instrlib>:"niDCPower Close.vi"("error in (no error)"=w391, "instrument handle"=w390) -> ("error out"=w383:errorcluster)  [unwired: 9 in]
          }
          frame Error {
            n131 = call <vilib>:"Clear Errors.vi"("error in (no error)"=w394) -> ("error out"=w401:errorcluster)  [unwired: 5 in, 1 out]
            n132 = Unbundle By Name(w394) -> ("source"=w393:string)
            n133 = call <instrlib>:"niSwitch Close.vi"("error in (no error)"=w401, "instrument handle"=w403) -> ("error out"=w402:errorcluster)  [unwired: 9 in]
            n134 = call <instrlib>:"niDMM Close.vi"("error in (no error)"=w402, "instrument handle"=w400) -> ("error out"=w397:errorcluster)  [unwired: 9 in]
            n135 = call <instrlib>:"niDCPower Abort With Channels.vi"("error in (no error)"=w397, "channel name"=w407, "instrument handle"=w410) -> ("error out"=w398:errorcluster, "instrument handle out"=w399:refnum<k15>)  [unwired: 7 in]
            n136 = call <instrlib>:"niDCPower Close.vi"("error in (no error)"=w398, "instrument handle"=w399) -> ("error out"=w411:errorcluster)  [unwired: 9 in]
            n137 = Concatenate Strings("Error occured during Measurement" ("message"), "\r", w393) -> (w392:string)
            n138 = call <instrlib>:"niDCPower Abort With Channels.vi"("error in (no error)"=w411, "channel name"=w406, "instrument handle"=w408) -> ("error out"=w413:errorcluster, "instrument handle out"=w412:refnum<k15>)  [unwired: 7 in]
            n139 = Bundle By Name(cluster=w405, "measurement results.Status"=w392) -> (w404:T3)
            n140 = call <instrlib>:"niDCPower Close.vi"("error in (no error)"=w413, "instrument handle"=w412) -> ("error out"=w409:errorcluster)  [unwired: 9 in]
          }
        }
      }
    }
  }
  "error out" <- w16
  "measure call context out" <- w17
  n141 = Unbundle By Name(w15) -> ("measurement results.Status"=w13:string, "Source Voltage-out"=w12:dbl[], "Source Current - out"=w11:dbl[], "Load Voltage-out"=w10:dbl[], "Load Current - out"=w9:dbl[])
  n142 = Bundle By Name(cluster=T1 {"Status"="Empty", "Source voltages"=[0.0], "Load voltages"=[0.0], "Source Current"=[0.0], "Load Current"=[0.0]} ("measurement results"), "Status"=w13, "Source voltages"=w12, "Source Current"=w11, "Load voltages"=w10, "Load Current"=w9) -> (→"measurement results":T1)
